vi "daemon.vi"(8 "stop":refnum<user-event>, 9 "Tags":map{string, string}(c390), 10 "Channel Name":string, 11 "Nominal Streaming in":refnum<class "Stream.lvclass">) -> ()   [LabVIEW 2020]
uses:
  Stream/Stream.lvclass
  Channel/Channel.lvclass
panel:
  out "Waveform Graph":waveform(dbl)(graph)
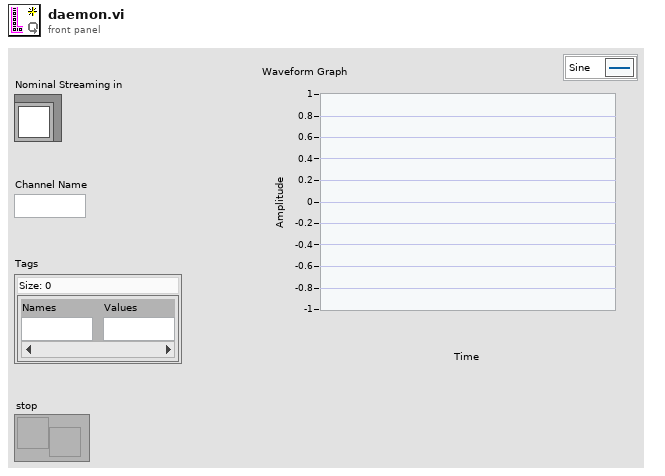
[diagram p1: front panel]
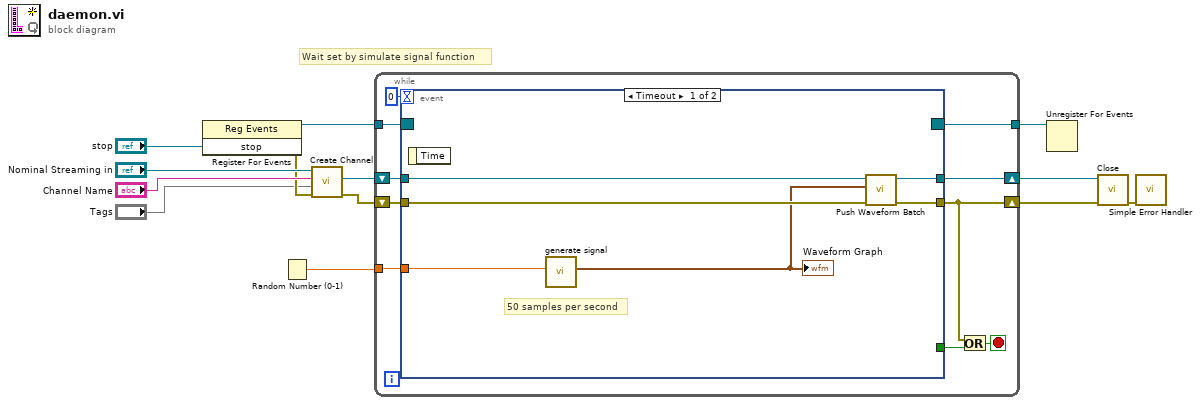
[diagram p0: block diagram]
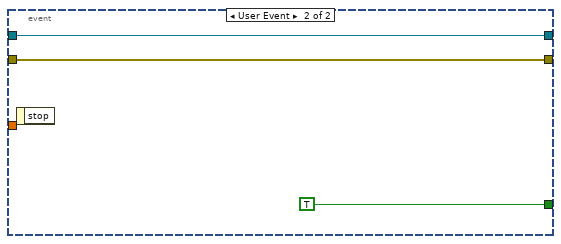
[diagram p2: hidden frame]
diagram:
  # "Wait set by simulate signal function"
  n1 = register-events("stop") -> (reference out=w6:refnum<event-registration>, error out=w5:errorcluster)  [unwired: 2 in]
  n2 = Random Number (0-1)() -> (number: 0 to 1=w1:dbl)
  n3 = call "Create Channel.vi"("error in (no error)"=w5, "Tags"="Tags", "Channel Name"="Channel Name", "Nominal Streaming in"="Nominal Streaming in") -> ("error out"=w9:errorcluster, "Channel"=w11:refnum<class "Channel.lvclass">)  [unwired: 5 in, 1 out]
  n4 = while {
    shift-right: [w22] -> w10
    shift-left: w11 -> [w23]
    shift-right: [w15] -> w8
    shift-left: w9 -> [w21]
    tunnel: [w19] -> w7
    tunnel: w6 -> [w18]
    tunnel: w1 -> [w14]
    stop <- w16 stop-if-true
    n5 = event shown="[0] Timeout" {
      selector: w18 -> [_ _]
      dyn-events: [_ _] -> w19
      timeout: 0 -> [_ _]
      tunnel: w23 -> [w29 w32]
      tunnel: [w28 w32] -> w22
      tunnel: w21 -> [w27 w31]
      tunnel: [w26 w31] -> w15
      tunnel: [_ TRUE] -> w17
      tunnel: w14 -> [w24 _]
      event Timeout {
        # "50 samples per second"
        n6 = event-data() -> ()  [unwired: 1 in, 1 out]
        n7 = call "generate signal.vi"("Phase"=w24) -> ("Waveform"=w25:waveform(dbl))  [unwired: 10 in]
        "Waveform Graph" <- w25
        n8 = call "Push Waveform Batch.vi"("error in (no error)"=w27, "Waveform"=w25, "Channel in"=w29) -> ("error out"=w26:errorcluster, "Channel out"=w28:refnum<class "Channel.lvclass">)  [unwired: 7 in]
      }
      event User Event {
        n9 = event-data() -> ()  [unwired: 1 in, 1 out]
      }
    }
    n10 = Or(x=w15, y=w17) -> (x .or. y?=w16:bool)
  }
  n11 = Unregister For Events(event registration refnum=w7) -> ()  [unwired: 1 in, 1 out]
  n12 = call "Close.vi"("error in (no error)"=w8, "Channel in"=w10) -> ("error out"=w2:errorcluster)  [unwired: 9 in]
  n13 = call <vilib>:"Simple Error Handler.vi"("error in (no error)"=w2) -> ()  [unwired: 4 in, 5 out]
